vi "Init MCP.vi"(8 "error in (no error)":errorcluster, 11 "Data Cluster in":T1) -> (0 "error out":errorcluster, 3 "Data Cluster out":T1)   [LabVIEW 2025, in "Scripting Server.lvlib"]
uses:
  Scripting Server.lvlib
  Module Data--cluster.ctl
  Config Data.ctl
  open_vi.vi
  create_project.vi
  get_allowed_paths.vi
  get_structure_diagram.vi
  get_loop_iteration_terminal.vi
  show_conditional_terminal.vi
  get_loop_conditional_terminal.vi
  get_object_help.vi
  connect_to_pane.vi
  add_subvi.vi
  set_value.vi
  save_vi.vi
  delete_object.vi
  enclose_selection.vi
  rename_object.vi
  add_to_selection.vi
  remove_from_selection.vi
  clear_selection_list.vi
  run_vi.vi
  create_control.vi
  cleanup_vi.vi
  get_vi_error_list.vi
  get_object_terminals.vi
  connect_objects.vi
  add_object.vi
  new_vi.vi
  <vilib>/jgoebel/LabVIEW MCP Server SDK/MCP Server.lvlibp
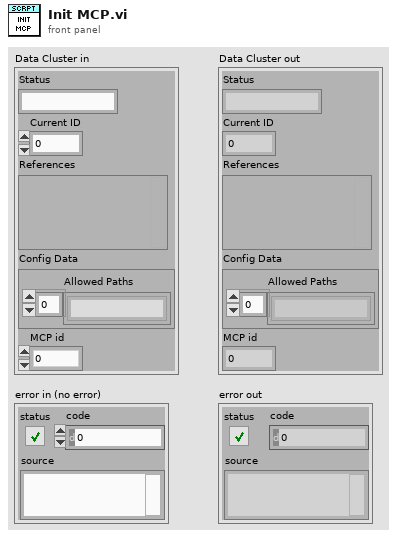
[diagram p1: front panel]
types:
  T1 = typedef "Scripting Server.lvlib/Module Data--cluster.ctl" = cluster{"Status":string, "Current ID":i32, "References":variant, "Config Data":T2, "MCP id":i32}
  T2 = typedef "Scripting Server.lvlib/Config Data.ctl" = cluster{"Allowed Paths":string[]}
  T3 = typedef "MCP Server.lvlibp/User Events.ctl" = cluster{"onError":refnum<user-event>, "onLog":refnum<user-event>, "onConnect":refnum<user-event>, "onToolsList":refnum<user-event>, "onToolsCall":refnum<user-event>, "onNotification":refnum<user-event>, "onTool":refnum<user-event>, "onRpc":refnum<user-event>}
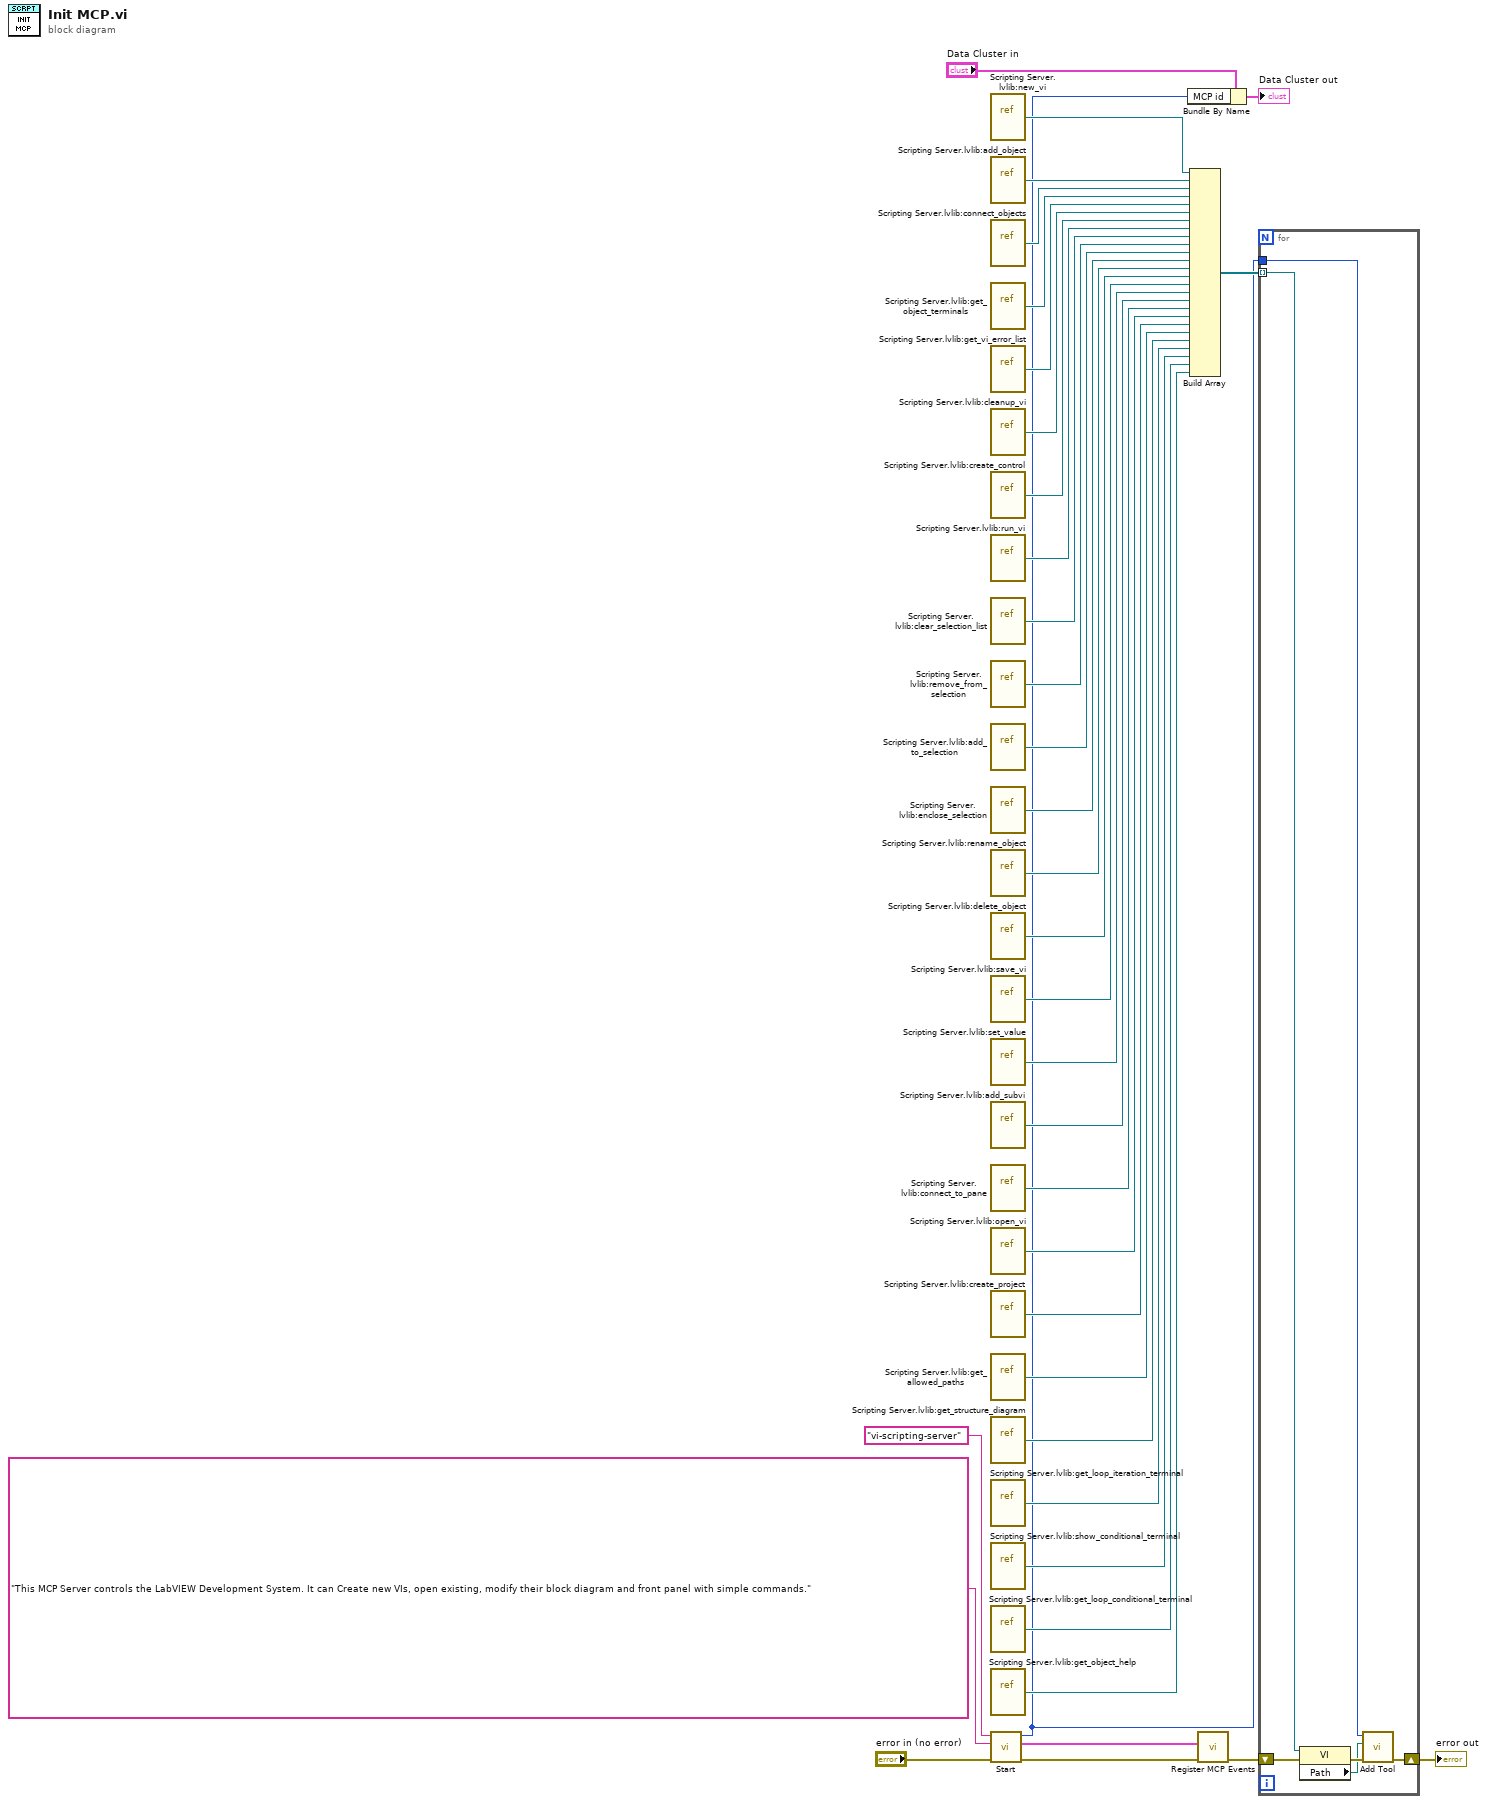
[diagram p0: block diagram]
diagram:
  n1 = vi-ref "Scripting Server.lvlib:new_vi.vi"() -> (w28:refnum<vi>)
  n2 = vi-ref "Scripting Server.lvlib:add_object.vi"() -> (w27:refnum<vi>)
  n3 = vi-ref "Scripting Server.lvlib:connect_objects.vi"() -> (w26:refnum<vi>)
  n4 = vi-ref "Scripting Server.lvlib:get_object_terminals.vi"() -> (w25:refnum<vi>)
  n5 = vi-ref "Scripting Server.lvlib:get_vi_error_list.vi"() -> (w24:refnum<vi>)
  n6 = vi-ref "Scripting Server.lvlib:cleanup_vi.vi"() -> (w23:refnum<vi>)
  n7 = vi-ref "Scripting Server.lvlib:create_control.vi"() -> (w22:refnum<vi>)
  n8 = vi-ref "Scripting Server.lvlib:run_vi.vi"() -> (w21:refnum<vi>)
  n9 = vi-ref "Scripting Server.lvlib:clear_selection_list.vi"() -> (w20:refnum<vi>)
  n10 = vi-ref "Scripting Server.lvlib:remove_from_selection.vi"() -> (w19:refnum<vi>)
  n11 = vi-ref "Scripting Server.lvlib:add_to_selection.vi"() -> (w18:refnum<vi>)
  n12 = vi-ref "Scripting Server.lvlib:enclose_selection.vi"() -> (w16:refnum<vi>)
  n13 = vi-ref "Scripting Server.lvlib:rename_object.vi"() -> (w17:refnum<vi>)
  n14 = vi-ref "Scripting Server.lvlib:delete_object.vi"() -> (w15:refnum<vi>)
  n15 = vi-ref "Scripting Server.lvlib:save_vi.vi"() -> (w14:refnum<vi>)
  n16 = vi-ref "Scripting Server.lvlib:set_value.vi"() -> (w13:refnum<vi>)
  n17 = vi-ref "Scripting Server.lvlib:add_subvi.vi"() -> (w12:refnum<vi>)
  n18 = vi-ref "Scripting Server.lvlib:connect_to_pane.vi"() -> (w11:refnum<vi>)
  n19 = vi-ref "Scripting Server.lvlib:open_vi.vi"() -> (w10:refnum<vi>)
  n20 = vi-ref "Scripting Server.lvlib:create_project.vi"() -> (w9:refnum<vi>)
  n21 = vi-ref "Scripting Server.lvlib:get_allowed_paths.vi"() -> (w8:refnum<vi>)
  n22 = vi-ref "Scripting Server.lvlib:get_structure_diagram.vi"() -> (w7:refnum<vi>)
  n23 = vi-ref "Scripting Server.lvlib:get_loop_iteration_terminal.vi"() -> (w6:refnum<vi>)
  n24 = vi-ref "Scripting Server.lvlib:show_conditional_terminal.vi"() -> (w5:refnum<vi>)
  n25 = vi-ref "Scripting Server.lvlib:get_loop_conditional_terminal.vi"() -> (w4:refnum<vi>)
  n26 = vi-ref "Scripting Server.lvlib:get_object_help.vi"() -> (w3:refnum<vi>)
  n27 = call <vilib>:"Start.vi"("error in (no error)"="error in (no error)", "Description"="This MCP Server controls the LabVIEW Development System. It can Create new VIs, open existing, modify their block diagram and front panel with simple commands.", "Name"="vi-scripting-server") -> ("error out"=w32:errorcluster, "User Events"=w30:T3, "id out"=w1:i32)  [unwired: 6 in]
  n28 = Bundle By Name(cluster="Data Cluster in", "MCP id"=w1) -> (→"Data Cluster out":T1)
  n29 = Build Array(w28, w27, w26, w25, w24, w23, w22, w21, w20, w19, w18, w16, w17, w15, w14, w13, w12, w11, w10, w9, w8, w7, w6, w5, w4, w3) -> (w2:refnum<vi>[])
  n30 = call "Register MCP Events.vi"("error in"=w32, "User Events"=w30) -> ("error out"=w31:errorcluster)  [unwired: 9 in]
  n31 = for {
    shift-right: [w42] -> w29
    shift-left: w31 -> [w43]
    tunnel: w2 -> [w40] mode=indexing
    tunnel: w1 -> [w38]
    n32 = property class="VI"(reference=w40, error in=w43) -> (error out=w41:errorcluster, "Path"=w39:path)  [unwired: 1 out]
    n33 = call <vilib>:"Add Tool.vi"("error in (no error)"=w41, "vi path"=w39, "id"=w38) -> ("error out"=w42:errorcluster)  [unwired: 7 in, 1 out]
  }
  "error out" <- w29
